vi "Set Connector Pane State.vi"(8 "error in (no error)":errorcluster, 10 "callers adapt? (true)":bool=TRUE, 11 "PPL in":refnum<class "NI_AB_API_DPPL.lvclass">) -> (0 "error out":errorcluster, 3 "PPL out":refnum<class "NI_AB_API_DPPL.lvclass">)   [LabVIEW 2020, in "NI_AB_API_DPPL.lvclass"]
uses:
  <vilib>/AppBuilder/AB_API/DPPL/NI_AB_API_DPPL.lvclass
  <vilib>/AppBuilder/AB_API/DPPL/NI_AB_API_DPPL.lvclass/NI_AB_API_DPPL.ctl
  <vilib>/AppBuilder/AB_API/PPL/NI_AB_API_PPL.lvclass
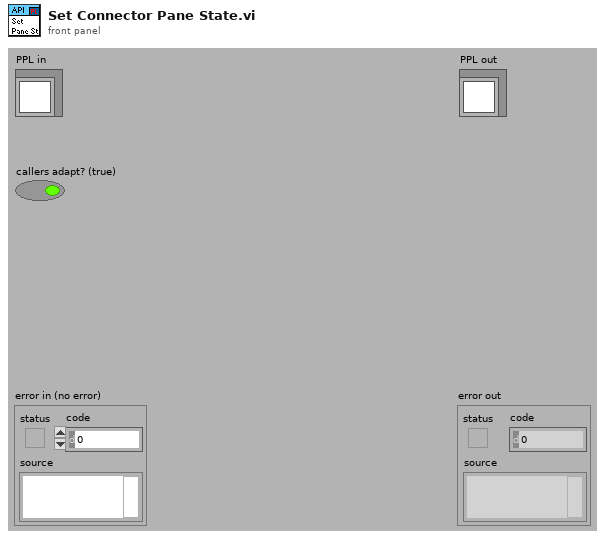
[diagram p1: front panel]
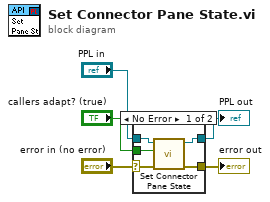
[diagram p0: block diagram]
diagram:
  n1 = case shown="No Error" "error in (no error)" {
    selector: "error in (no error)" -> [w7 w12]
    tunnel: [w8 w12] -> w3
    tunnel: [w9 w11] -> w4
    tunnel: "PPL in" -> [w10 w11]
    tunnel: "callers adapt? (true)" -> [w6 _]
    frame No Error {
      n2 = call-parent "Set Connector Pane State.vi"("error in (no error)"=w7, "callers adapt? (true)"=w6, "PPL in"=w10) -> ("error out"=w8:errorcluster, "PPL out"=w9:refnum<class "NI_AB_API_DPPL.lvclass">)  [unwired: 7 in]
    }
    frame Error {
    }
  }
  "error out" <- w3
  "PPL out" <- w4
